vi "Histogram2D_Automatic.vi"(4 "Properties":T2={"Normalize"=FALSE, "Colormap"={"Map"=enum."Automatic", "Value Min"=nan, "Value Max"=nan, "Scaling"=enum."Default", "Reverse"=FALSE}, "Display"={"Alpha"=nan, "Z Order"=nan}}, 5 "Y Bins":i32=-1, 6 "Data Range":T1={"X Min"=nan, "X Max"=nan, "Y Min"=nan, "Y Max"=nan}, 7 "X Bins":i32=-1, 8 "error in (no error)":errorcluster, 9 "Y Data":dbl[](array[numeric]), 10 "X Data":dbl[](array[numeric]), 11 "Plot ID":T7 format="%x") -> (0 "error out":errorcluster, 3 "Plot ID Out":T7 format="%x")   [LabVIEW 2013, in "Advanced Plotting Toolkit.lvlib"]
doc: "Create a 2D histogram from two data sets in X and Y, visualized as a 2D plane of colored patches."
uses:
  Advanced Plotting Toolkit.lvlib
  typedefs/PlotID.ctl
  Histogram2DProperties.ctl
  properties/Colormap.ctl
  properties/Colormap_Map.ctl
  properties/Colormap_Scaling.ctl
  properties/Display.ctl
  Histogram2DRange.ctl
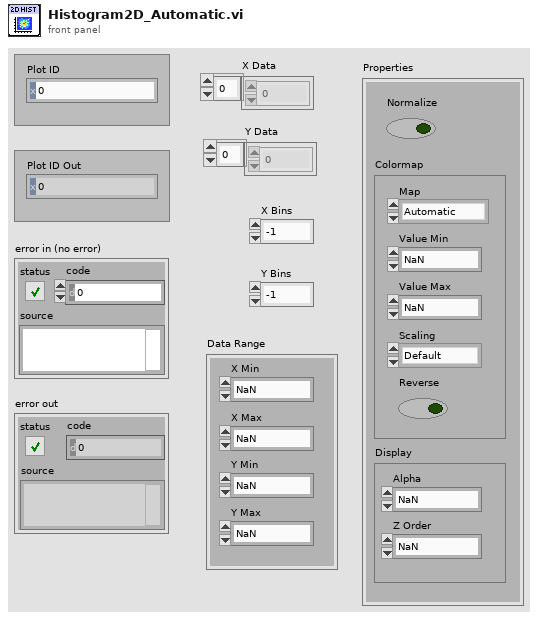
[diagram p1: front panel]
types:
  T1 = typedef "Advanced Plotting Toolkit.lvlib/Histogram2DRange.ctl" = cluster{"X Min":dbl, "X Max":dbl, "Y Min":dbl, "Y Max":dbl}
  T2 = typedef "Advanced Plotting Toolkit.lvlib/Histogram2DProperties.ctl" = cluster{"Normalize":bool, "Colormap":T3, "Display":T6}
  T3 = typedef "Advanced Plotting Toolkit.lvlib/Colormap.ctl" = cluster{"Map":T4, "Value Min":dbl, "Value Max":dbl, "Scaling":T5, "Reverse":bool}
  T4 = typedef "Advanced Plotting Toolkit.lvlib/Colormap_Map.ctl" = enum16{"Automatic", "Rainbow", "Hot and Cold", "White-Black", "White-Blue", "White-Green", "White-Red", "Fire", "Water", "Earth", "Air", "Pastel", "Banded", "Stepped"}
  T5 = typedef "Advanced Plotting Toolkit.lvlib/Colormap_Scaling.ctl" = enum16{"Default"}
  T6 = typedef "Advanced Plotting Toolkit.lvlib/Display.ctl" = cluster{"Alpha":dbl, "Z Order":dbl}
  T7 = typedef "Advanced Plotting Toolkit.lvlib/PlotID.ctl" = i32
  T8 = typedef "Advanced Plotting Toolkit.lvlib/KeyValue.ctl" = cluster{"Key":string, "Value":string}
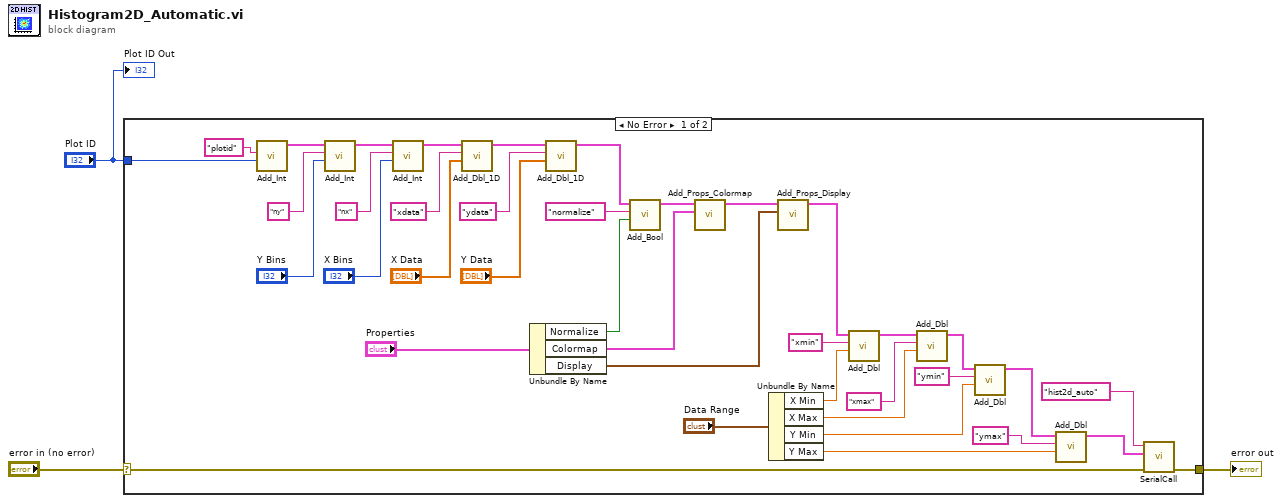
[diagram p0: block diagram]
diagram:
  n1 = case shown="No Error" "error in (no error)" {
    selector: "error in (no error)" -> [w34 w43]
    tunnel: "Plot ID" -> [w42 _]
    tunnel: [w33 w43] -> w1
    frame No Error {
      n2 = call "Add_Int.vi"("Value"=w42, "Key"="plotid") -> ("Keyword Array Out"=w23:T8[])  [unwired: 9 in]
      n3 = call "Add_Int.vi"("Value"="Y Bins", "Key"="ny", "Keyword Array"=w23) -> ("Keyword Array Out"=w22:T8[])  [unwired: 8 in]
      n4 = call "Add_Int.vi"("Value"="X Bins", "Key"="nx", "Keyword Array"=w22) -> ("Keyword Array Out"=w38:T8[])  [unwired: 8 in]
      n5 = call "Add_Dbl_1D.vi"("Value"="X Data", "Key"="xdata", "Keyword Array"=w38) -> ("Keyword Array Out"=w21:T8[])  [unwired: 8 in]
      n6 = Unbundle By Name("Properties") -> ("Normalize"=w15:bool, "Colormap"=w6:T3, "Display"=w5:T6)
      n7 = call "Add_Dbl_1D.vi"("Value"="Y Data", "Key"="ydata", "Keyword Array"=w21) -> ("Keyword Array Out"=w16:T8[])  [unwired: 8 in]
      n8 = call "Add_Bool.vi"("Value"=w15, "Key"="normalize", "Keyword Array"=w16) -> ("Keyword Array Out"=w4:T8[])  [unwired: 8 in]
      n9 = call "Add_Props_Colormap.vi"("Colormap"=w6, "Keyword Array"=w4) -> ("Keyword Array Out"=w9:T8[])  [unwired: 9 in]
      n10 = Unbundle By Name("Data Range") -> ("X Min"=w13:dbl, "X Max"=w12:dbl, "Y Min"=w11:dbl, "Y Max"=w10:dbl)
      n11 = call "Add_Props_Display.vi"("Display"=w5, "Keyword Array"=w9) -> ("Keyword Array Out"=w8:T8[])  [unwired: 9 in]
      n12 = call "Add_Dbl.vi"("Value"=w13, "Key"="xmin", "Keyword Array"=w8) -> ("Keyword Array Out"=w28:T8[])  [unwired: 8 in]
      n13 = call "Add_Dbl.vi"("Value"=w12, "Key"="xmax", "Keyword Array"=w28) -> ("Keyword Array Out"=w27:T8[])  [unwired: 8 in]
      n14 = call "Add_Dbl.vi"("Value"=w11, "Key"="ymin", "Keyword Array"=w27) -> ("Keyword Array Out"=w26:T8[])  [unwired: 8 in]
      n15 = call "Add_Dbl.vi"("Value"=w10, "Key"="ymax", "Keyword Array"=w26) -> ("Keyword Array Out"=w7:T8[])  [unwired: 8 in]
      n16 = call "SerialCall.vi"("error in (no error)"=w34, "data"=w7, "Resource"="hist2d_auto") -> ("error out"=w33:errorcluster)  [unwired: 7 in, 1 out]
    }
    frame Error {
    }
  }
  "error out" <- w1
  "Plot ID Out" <- "Plot ID"
